vi "Main.vi"() -> ()   [LabVIEW 2021]
doc: "Use this template to build a simple state machine design pattern. Each state executes code and determines which state to transition to."
uses:
  controls/State.ctl
  controls/Data.ctl
  <vilib>/DAQmx/configure/timing.llb/DAQmx Timing (Sample Clock).vi
  <vilib>/DAQmx/create/channels.llb/DAQmx Create Channel (AI-Voltage-Basic).vi
  <vilib>/DAQmx/read.llb/DAQmx Read (Analog Wfm 1Chan NSamp).vi
  <vilib>/Waveform/WDTOps.llb/WDT Append Waveforms DBL.vi
panel:
  in  "stop measure":bool
  in  "Measure Init":bool
  in  "Number of Samples":i32=100
  in  "Sample Rate":dbl=1000.0
  in  "Sample Clock Source":tag="OnboardClock"
  in  "Terminal Configuration":i32(ring)=-1 items=["default"=-1, "RSE"=10083, "NRSE"=10078, "Differential"=10106, "Pseudodifferential"=12529]
  in  "Max Voltage":dbl=5.0
  in  "Min Voltage":dbl=-5.0
  in  "Physical Channel":tag="Dev1/ai0"
  out "Waveform Graph":dbl[](graph)
  in  "Write to TDMS":bool
  in  "Start measuring":bool
  in  "Exit":bool
  # "These controls have associated \"Value Changed\" events configured in the Event Structure on the diagram.\n\nReplace them (and reconfigure the Event Structure) with the controls you need for your application."
  # "This template is for the Simple State Machine design pattern.\n\nSee the block diagram for more information on how to use this template."
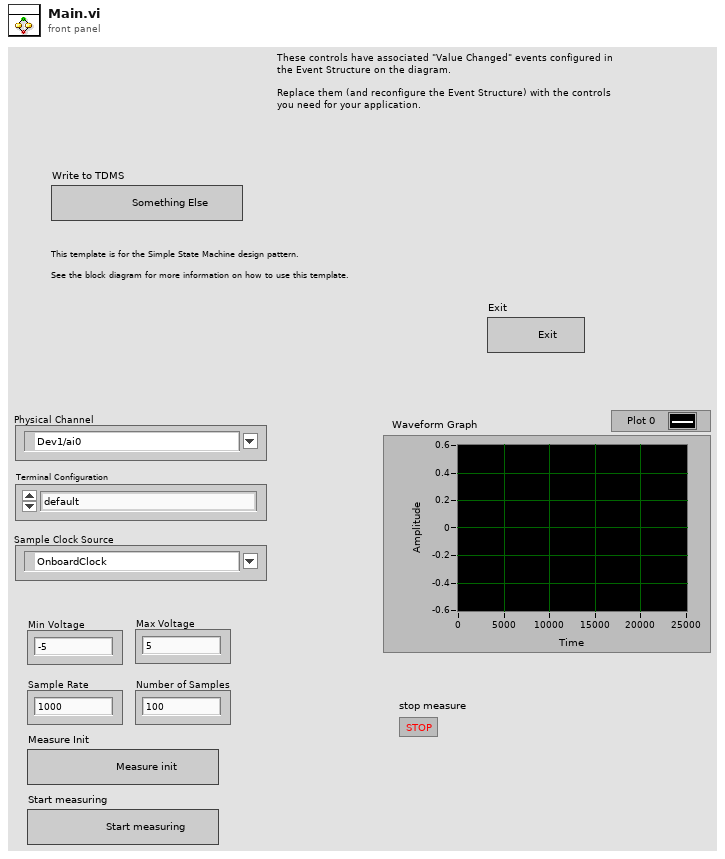
[diagram p1: front panel]
types:
  T1 = typedef "Data.ctl" = cluster{"DAQmx Task Name":refnum<k21>, "Mes running":bool, "Waveform":waveform(dbl)}
  T2 = typedef "State.ctl" = enum16{"Initialize", "Wait for Event", "Mesurement init", "START measure", "Measuring", "STOP measure", "Data analyze", "TDMS write", "Error", "Exit"}
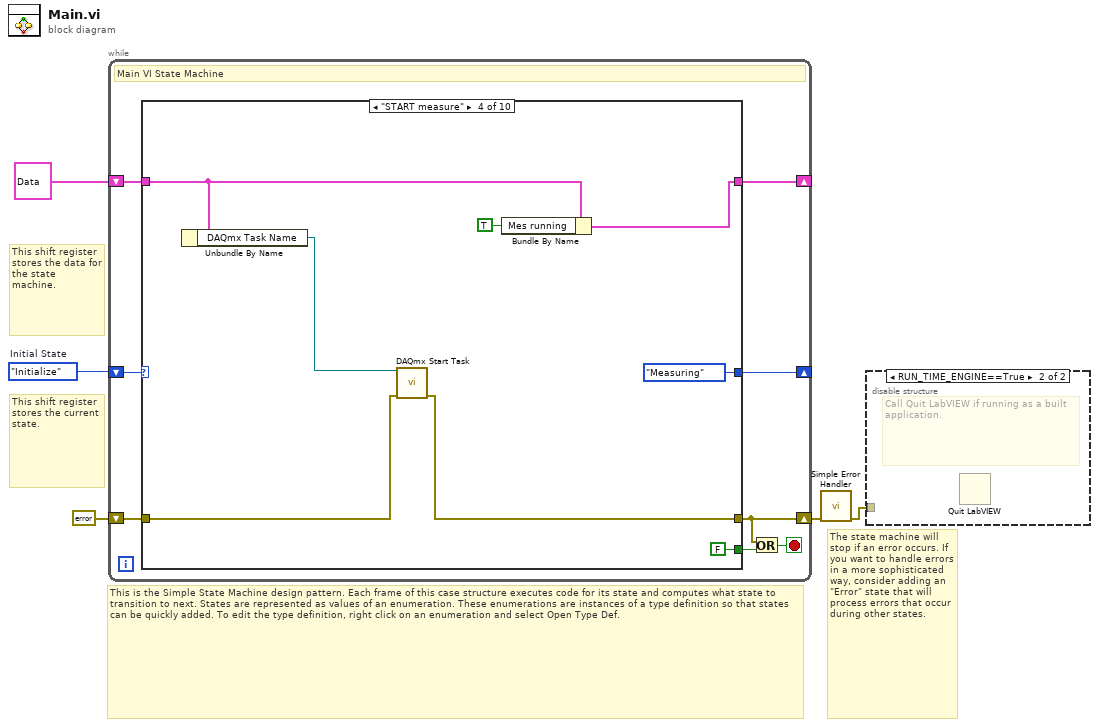
[diagram p0: block diagram]
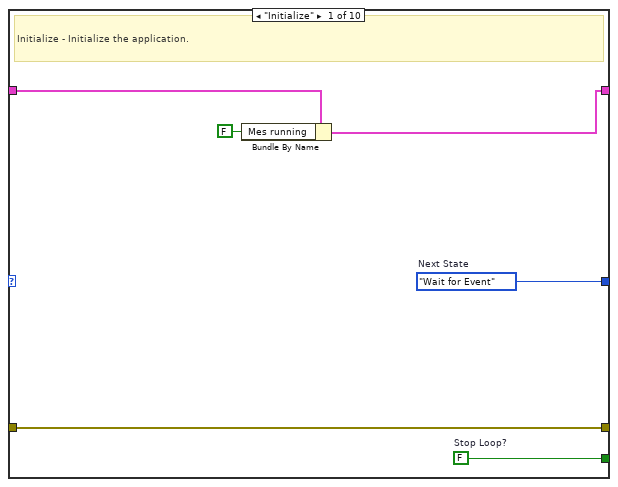
[diagram p3: hidden frame]
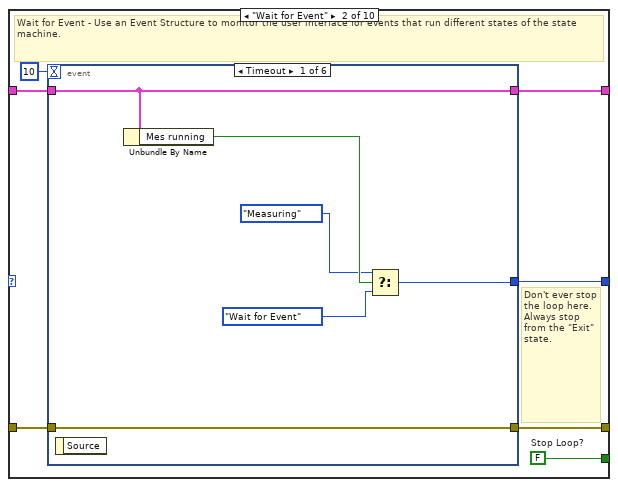
[diagram p4: hidden frame]
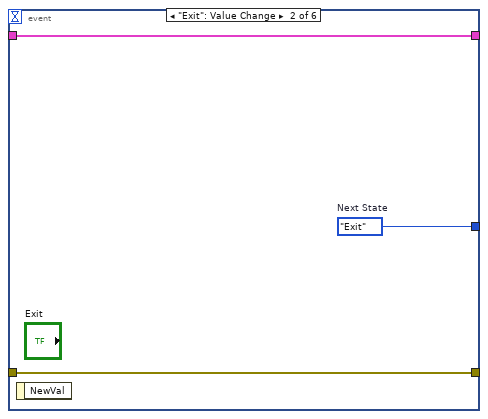
[diagram p5: hidden frame]
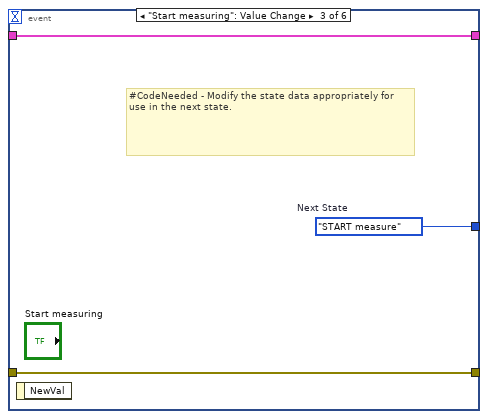
[diagram p6: hidden frame]
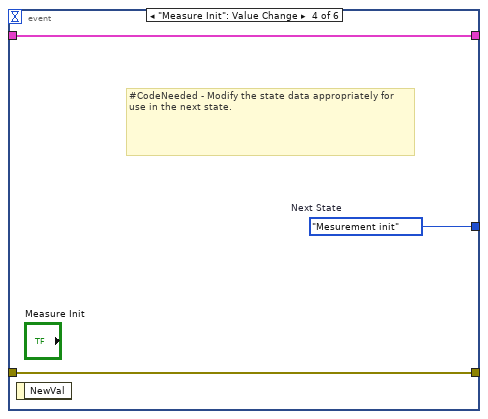
[diagram p7: hidden frame]
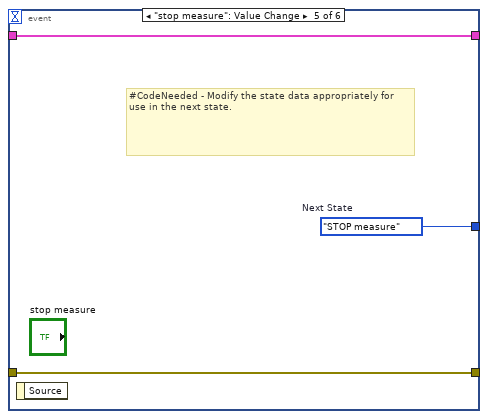
[diagram p8: hidden frame]
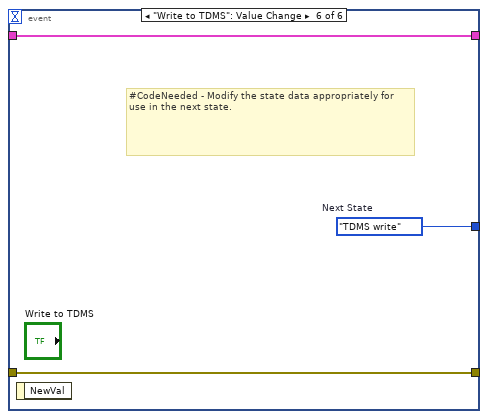
[diagram p9: hidden frame]
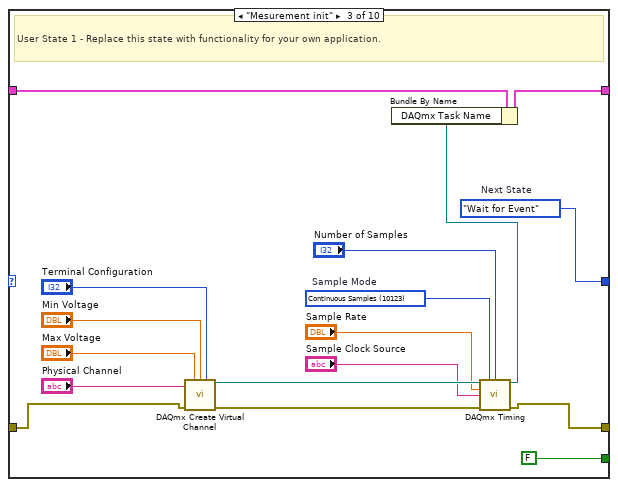
[diagram p10: hidden frame]
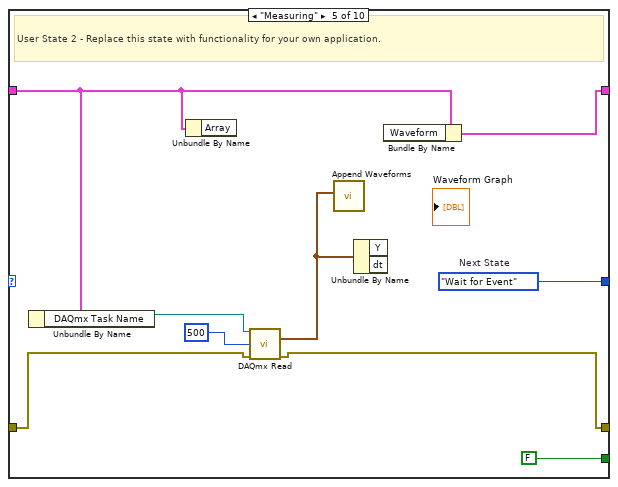
[diagram p11: hidden frame]
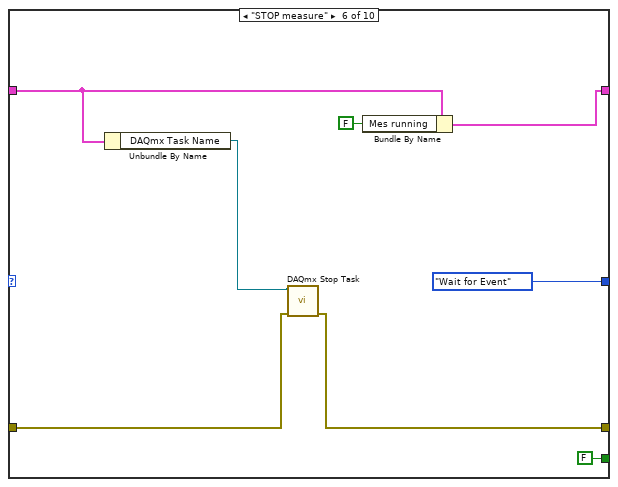
[diagram p12: hidden frame]
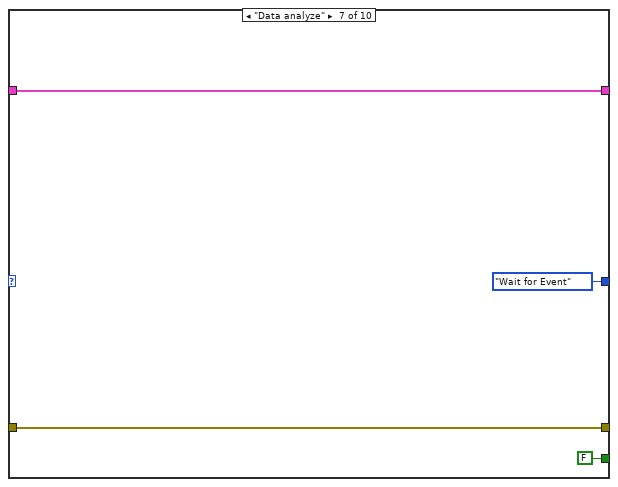
[diagram p13: hidden frame]
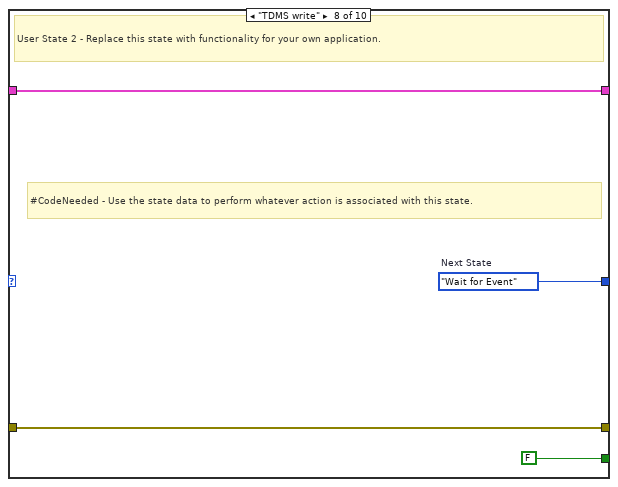
[diagram p14: hidden frame]
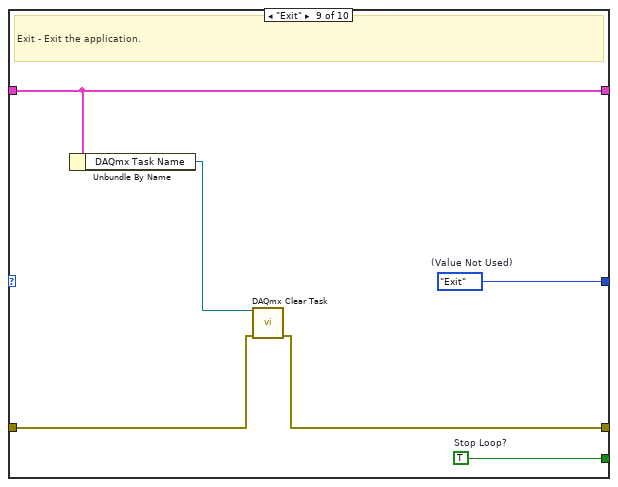
[diagram p15: hidden frame]
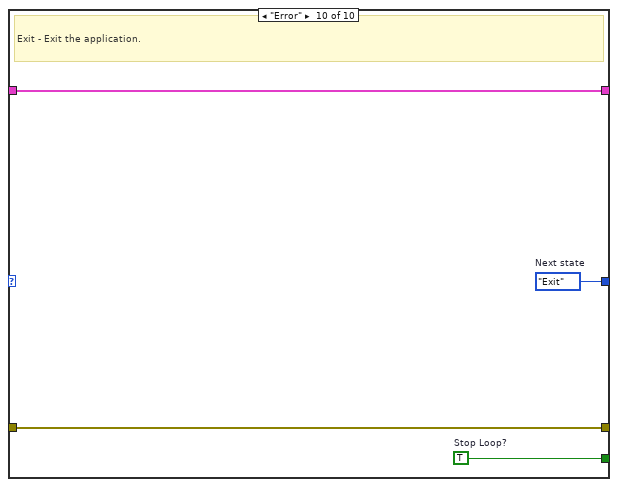
[diagram p16: hidden frame]
diagram:
  w1 = State."Initialize"  # Initial State
  # "The state machine will stop if an error occurs. If you want to handle errors in a more sophisticated way, consider adding an \"Error\" state that will process errors that occur during other states."
  # "This shift register stores the data for the state machine."
  # "This is the Simple State Machine design pattern. Each frame of this case structure executes code for its state and computes what state to transition to next. States are represented as values of an enumeration. These enumerations are instances of a type definition so that states can be quickly added. To edit the type definition, right click on an enumeration and select Open Type Def."
  # "This shift register stores the current state."
  n1 = while {
    shift-right: [w12] -> _
    shift-left: w1 -> [w13]
    shift-right: [w10] -> _
    shift-left: T1 {"DAQmx Task Name"="", "Mes running"=FALSE, "Waveform"={"t0"=timestamp(0 s since 1904-01-01), "dt"=1.0, "Y"=[]}} ("Data") -> [w11]
    shift-right: [w6] -> w3
    shift-left: errorcluster {"status"=FALSE, "code"=0, "source"=""} ("error constant") -> [w9]
    stop <- w7 stop-if-true
    # "Main VI State Machine"
    n2 = case shown="\"START measure\"" w13 {
      tunnel: [w19 w26 w64 State."Measuring" ("Next state") w81 State."Wait for Event" ("Next state") State."Wait for Event" ("Next state") w97 w103 w107] -> w12
      tunnel: [w18 w25 FALSE ("Stop Loop?") FALSE ("Stop Loop?") FALSE ("Stop Loop?") FALSE ("Stop Loop?") FALSE ("Stop Loop?") FALSE ("Stop Loop?") w102 w105] -> w8
      tunnel: w11 -> [w16 w24 w62 w67 w75 w87 w93 w95 w99 w106]
      tunnel: [w15 w23 w61 w66 w76 w86 w93 w95 w99 w106] -> w10
      tunnel: w9 -> [w17 w22 w50 w72 w79 w83 w92 w94 w101 w104]
      tunnel: [w17 w21 w49 w71 w78 w82 w92 w94 w100 w104] -> w6
      frame "Initialize" {
        w18 = FALSE  # Stop Loop?
        w19 = State."Wait for Event"  # Next State
        # "Initialize - Initialize the application."
        n3 = Bundle By Name(cluster=w16, "Mes running"=FALSE) -> (w15:T1)
      }
      frame "Wait for Event" {
        w25 = FALSE  # Stop Loop?
        # "Don't ever stop the loop here. Always stop from the \"Exit\" state."
        # "Wait for Event - Use an Event Structure to monitor the user interface for events that run different states of the state machine."
        n4 = event shown="[0] Timeout" {
          selector: _ -> [_ _ _ _ _ _]
          dyn-events: _ -> [_ _ _ _ _ _]
          timeout: 10 -> [_ _ _ _ _ _]
          tunnel: [w31 w35 w38 w41 w44 w47] -> w26
          tunnel: w24 -> [w30 w34 w36 w39 w42 w45]
          tunnel: [w30 w34 w36 w39 w42 w45] -> w23
          tunnel: w22 -> [w32 w33 w37 w40 w43 w46]
          tunnel: [w32 w33 w37 w40 w43 w46] -> w21
          event Timeout {
            n5 = event-data() -> ()  [unwired: 1 in, 1 out]
            n6 = Unbundle By Name(w30) -> ("Mes running"=w29:bool)
            n7 = Select(t=State."Measuring" ("Next State"), s=w29, f=State."Wait for Event" ("Next State")) -> (s? t:f=w31:T2)
          }
          event "Exit": Value Change {
            w35 = State."Exit"  # Next State
            n8 = event-data() -> ()  [unwired: 1 in, 1 out]
          }
          event "Start measuring": Value Change {
            w38 = State."START measure"  # Next State
            # "#CodeNeeded - Modify the state data appropriately for use in the next state."
            n9 = event-data() -> ()  [unwired: 1 in, 1 out]
          }
          event "Measure Init": Value Change {
            w41 = State."Mesurement init"  # Next State
            # "#CodeNeeded - Modify the state data appropriately for use in the next state."
            n10 = event-data() -> ()  [unwired: 1 in, 1 out]
          }
          event "stop measure": Value Change {
            w44 = State."STOP measure"  # Next State
            # "#CodeNeeded - Modify the state data appropriately for use in the next state."
            n11 = event-data() -> ()  [unwired: 1 in, 1 out]
          }
          event "Write to TDMS": Value Change {
            w47 = State."TDMS write"  # Next State
            # "#CodeNeeded - Modify the state data appropriately for use in the next state."
            n12 = event-data() -> ()  [unwired: 1 in, 1 out]
          }
        }
      }
      frame "Mesurement init" {
        w60 = 10123 items=["Finite Samples"=10178, "Continuous Samples"=10123, "Hardware Timed Single Point"=12522]  # Sample Mode
        w64 = State."Wait for Event"  # Next State
        # "User State 1 - Replace this state with functionality for your own application."
        n13 = call-poly <vilib>:"DAQmx Create Virtual Channel.vi"("maximum value"="Max Voltage", "minimum value"="Min Voltage", "input terminal configuration"="Terminal Configuration", "physical channels"="Physical Channel", "error in"=w50) -> ("task out"=w58:refnum<k21>, "error out"=w59:errorcluster)  [unwired: 9 in]
        n14 = call-poly <vilib>:"DAQmx Timing.vi"("task/channels in"=w58, "sample mode"=w60, "samples per channel"="Number of Samples", "rate"="Sample Rate", "source"="Sample Clock Source", "error in"=w59) -> ("task out"=w48:refnum<k21>, "error out"=w49:errorcluster)  [unwired: 8 in]
        n15 = Bundle By Name(cluster=w62, "DAQmx Task Name"=w48) -> (w61:T1)
      }
      frame "START measure" {
        n16 = Unbundle By Name(w67) -> ("DAQmx Task Name"=w70:refnum<k21>)
        n17 = call <vilib>:"DAQmx Start Task.vi"("task/channels in"=w70, "error in"=w72) -> ("error out"=w71:errorcluster)  [unwired: 12 in, 1 out]
        n18 = Bundle By Name(cluster=w67, "Mes running"=TRUE) -> (w66:T1)
      }
      frame "Measuring" {
        w81 = State."Wait for Event"  # Next State
        # "User State 2 - Replace this state with functionality for your own application."
        n19 = Unbundle By Name(w75) -> ("DAQmx Task Name"=w77:refnum<k21>)
        n20 = Unbundle By Name(w75) -> ()  [unwired: 1 out]
        n21 = call-poly <vilib>:"DAQmx Read.vi"("task/channels in"=w77, "number of samples per channel"=500, "error in"=w79) -> ("data"=w73:waveform(dbl), "error out"=w78:errorcluster)  [unwired: 10 in, 1 out]
        n22 = call-poly <vilib>:"Append Waveforms.vi"("waveform B"=w73) -> ()  [unwired: 9 in, 2 out]
        n23 = Unbundle By Name(w73) -> ()  [unwired: 2 out]
        n24 = Bundle By Name(cluster=w75) -> (w76:T1)  [unwired: 1 in]
      }
      frame "STOP measure" {
        n25 = Unbundle By Name(w87) -> ("DAQmx Task Name"=w84:refnum<k21>)
        n26 = call <vilib>:"DAQmx Stop Task.vi"("task/channels in"=w84, "error in"=w83) -> ("error out"=w82:errorcluster)  [unwired: 12 in, 1 out]
        n27 = Bundle By Name(cluster=w87, "Mes running"=FALSE) -> (w86:T1)
      }
      frame "Data analyze" {
      }
      frame "TDMS write" {
        w97 = State."Wait for Event"  # Next State
        # "#CodeNeeded - Use the state data to perform whatever action is associated with this state."
        # "User State 2 - Replace this state with functionality for your own application."
      }
      frame "Exit" {
        w102 = TRUE  # Stop Loop?
        w103 = State."Exit"  # (Value Not Used)
        # "Exit - Exit the application."
        n28 = Unbundle By Name(w99) -> ("DAQmx Task Name"=w98:refnum<k21>)
        n29 = call <vilib>:"DAQmx Clear Task.vi"("task in"=w98, "error in"=w101) -> ("error out"=w100:errorcluster)  [unwired: 13 in]
      }
      frame "Error" {
        w105 = TRUE  # Stop Loop?
        w107 = State."Exit"  # Next state
        # "Exit - Exit the application."
      }
    }
    n30 = Or(x=w6, y=w8) -> (x .or. y?=w7:bool)
  }
  n31 = call <vilib>:"Simple Error Handler.vi"("error in (no error)"=w3) -> ("error out"=w2:errorcluster)  [unwired: 4 in, 4 out]
  n32 = disable-structure shown="RUN_TIME_ENGINE==True" {
    disable-tunnel: w2 -> [_ _]
    frame condition #0 (active) {
    }
    frame condition #1 {
      # "Call Quit LabVIEW if running as a built application."
      n33 = Quit LabVIEW() -> ()  [unwired: 1 in]
    }
  }
